vi "I2C_WriteReadMemoryBlock.vi"(8 "error in (no error)":errorcluster, 10 "MemoryAddress":u32, 11 "Bits":bool[](array[boolean])=[FALSE, FALSE, FALSE, FALSE, FALSE, FALSE, FALSE, FALSE]) -> (0 "error out":errorcluster)   [LabVIEW 2019]
doc: "Writes Bytes received from the Slave Device into the Read Memory block for the Host VI to access.\n\nVI Written By:\nPeter Fuller\nSenior Engineer\nplf Consulting, LLC\n617.699.2201"
uses:
  <vilib>/Utility/error.llb/Clear Errors.vi
  <vilib>/rvi/Emulation/niFpgaSctlEmulationGetInTimedLoop.vi
  <vilib>/rvi/Memory/Memory_Emulation/nirvimemoryEmulation.vi
  <vilib>/rvi/Memory/Memory_Emulation/nirvimemoryFastEmulation.vi
  <vilib>/rvi/DataTransferAndStorage/Container/Common/niFpgaContainerGetUniqueNameForEmu.vi
  <vilib>/rvi/Memory/Memory_Emulation/niFpgaMemoryEmulationCacheClearOnFirstRun.vi
  <vilib>/rvi/Memory/Memory_Emulation/nirvimemoryEmulationManagerCache_MakeExclusive.vi
  <vilib>/rvi/Memory/Memory_Emulation/niFpgaMemoryEmulationValidateCache.vi
  <vilib>/rvi/Memory/Memory_Emulation/nirvimemoryEmulationManagerCache_InsertValue.vi
  <vilib>/rvi/Memory/Memory_Emulation/nirvimemoryEmulationManagerCache_ReleaseExclusive.vi
  <vilib>/rvi/Memory/Memory_Emulation/nirvimemoryEmulationManagerCache_GetValue.vi
  <vilib>/rvi/Emulation/niFpgaEmulationIsFPGAContextNoSignature.vi
  <vilib>/rvi/Memory/Memory_Emulation/nirvimemoryEmulationManagerCache_SetValue.vi
  <vilib>/rvi/Emulation/niFpgaSctlEmulationResourceMgr.vi
  <vilib>/rvi/DataTransferAndStorage/Container/XNode/niFpgaContainer.xnode
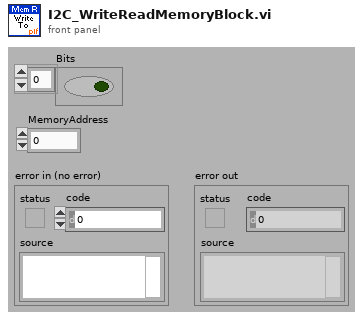
[diagram p1: front panel]
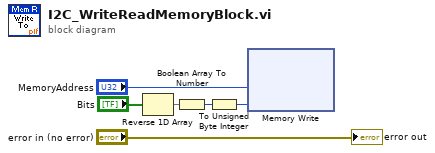
[diagram p0: block diagram]
diagram:
  n1 = Reverse 1D Array(array="Bits") -> (reversed array=w4:bool[])
  n2 = Boolean Array To Number(Boolean array=w4) -> (number=w3:u8)
  n3 = To Unsigned Byte Integer(number=w3) -> (unsigned 8bit integer=w2:u8)
  n4 = xnode ("Memory Write")("Address"="MemoryAddress", "Data"=w2) -> ()  [unwired: 1 in, 1 out]
  "error out" <- "error in (no error)"
